vi "Auton Rotation Control.vi"(0 "Feedback":dbl, 3 "PID gains":T1={"proportional gain (Kc)"=0.9, "integral time (Ti, min)"=0.06, "derivative time (Td, min)"=0.0} {"derivative time (Td, min)" format="%.5f"; "integral time (Ti, min)" format="%.5f"; "proportional gain (Kc)" format="%.5f"}, 9 "Setpoint":dbl) -> (14 "PID PWM 5 Output":dbl)   [LabVIEW 2011]
uses:
  Robot Global Data.vi
  <vilib>/addons/control/pid/pid.llb/PID (DBL).vi
  <vilib>/addons/control/pid/NI_PID_pid.lvlib
panel:
  out "Ramp":dbl=3.0
  in  "Down Rate":dbl=0.0275
  out "Ramping":bool
  out "Moving UP?":bool
  # "Up Rate\n.05"
  # "110\n120\n165\n165"
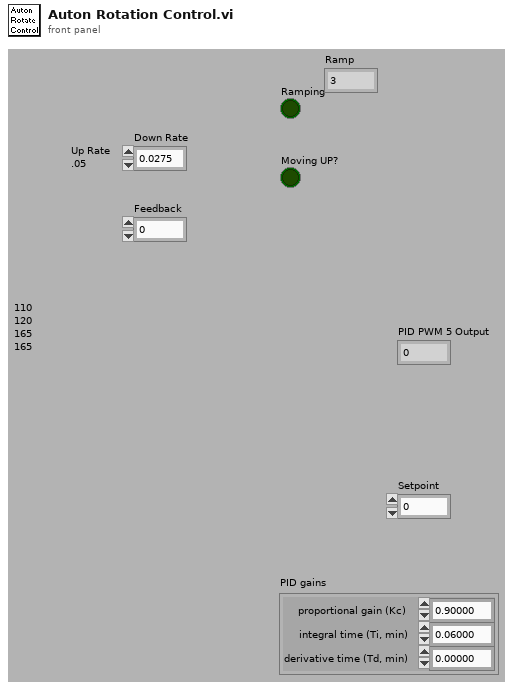
[diagram p1: front panel]
types:
  T1 = cluster{"proportional gain (Kc)":dbl, "integral time (Ti, min)":dbl, "derivative time (Td, min)":dbl}
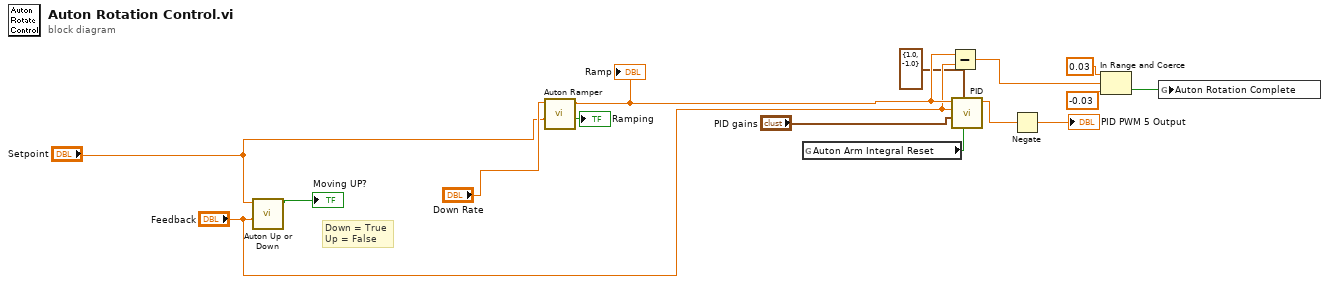
[diagram p0: block diagram]
diagram:
  # "Down = True\nUp = False"
  n1 = call "Auton Up or Down.vi"("Current Position (deg)"="Feedback", "Current Setpoint (deg)"="Setpoint") -> ("Moving UP?"=→"Moving UP?":bool)  [unwired: 9 out]
  n2 = call "Auton Ramper.vi"("Target Setpoint"="Setpoint", "Rate"="Down Rate") -> ("Ramping"=→"Ramping":bool, "Current Setpoint"=w8:dbl)  [unwired: 8 out]
  "Ramp" <- w8
  n3 = global read "Robot Global Data.vi" "Auton Arm Integral Reset"() -> (w13:bool)
  n4 = Subtract(x=w8, y="Feedback") -> (x-y=w11:dbl)
  n5 = call-poly <vilib>:"PID.vi"("reinitialize? (F)"=w13, "output range"=cluster{"output high":dbl, "output low":dbl} {"output high"=1.0, "output low"=-1.0}, "PID gains"="PID gains", "process variable"="Feedback", "setpoint"=w8) -> ("output"=w1:dbl)  [unwired: 1 in, 5 out]
  n6 = Negate(x=w1) -> (-x=→"PID PWM 5 Output":dbl)
  n7 = In Range and Coerce(upper limit=0.03, x=w11, lower limit=-0.03) -> (In Range?=w10:bool)  [unwired: 1 out]
  n8 = global write "Robot Global Data.vi" "Auton Rotation Complete"(w10) -> ()
